vi "Charakterystyki.vi"() -> ()   [LabVIEW 2020]
uses:
  <vilib>/addons/Digital Filter Design/Analysis.llb/DFD Plot Freq Response (Linear-Spaced).vi
  <vilib>/addons/Digital Filter Design/NI_DigFilterLicensed.lvlib
panel:
  in  "stop":bool
  out "Charakterystyka fazowa":cluster{"f0":dbl, "df":dbl, "values":dbl[]}[](graph)
  out "Charakterystyka amplitudowa":cluster{"f0":dbl, "df":dbl, "values":dbl[]}[](graph)
  out "Charakterystyka fazowa":cluster{"f0":dbl, "df":dbl, "values":dbl[]}[](graph)
  out "Charakterystyka amplitudowa":cluster{"f0":dbl, "df":dbl, "values":dbl[]}[](graph)
  out "Charakterystyka fazowa":cluster{"f0":dbl, "df":dbl, "values":dbl[]}[](graph)
  out "Charakterystyka amplitudowa":cluster{"f0":dbl, "df":dbl, "values":dbl[]}[](graph)
  # "Filtr Butterwortha"
  # "Filtr Czebyszewa"
  # "Filtr Bessela"
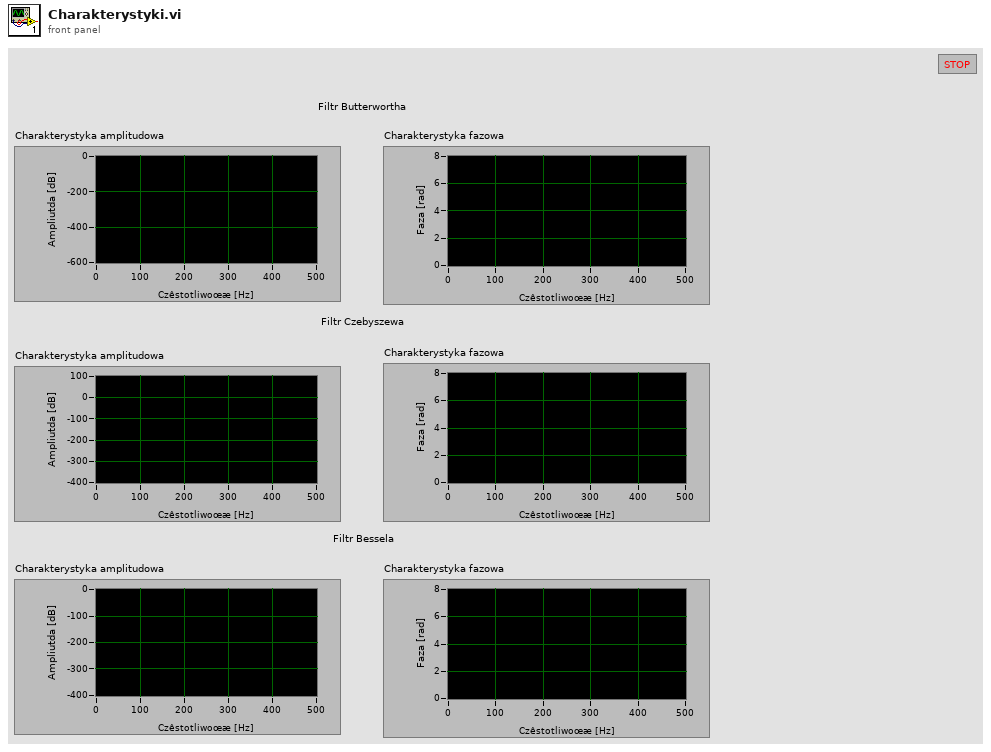
[diagram p1: front panel]
types:
  T1 = enum16{"Lowpass", "Highpass", "Bandpass", "Bandstop"}
  T2 = typedef "NI_DigFilterLicensed.lvlib/DFD Filter Obj.ctl" = cluster{"mSRate_Fs":dbl, "mSRate_Version":string, "mSRate_Comments":string, "mSRate_OrgCoef":T3, "mSRate_CurCoef":T3, "mSRate_Quantized?":bool, "mSRate_QCoef":T3, "mSRate_QSettings":T5[], "mSRate_Order":i32, "mSRate_Scaling":cluster{"mSRate_ScaleByPowerOf2?":bool, "mSRate_ScaleType":T7}}
  T3 = typedef "NI_DigFilterLicensed.lvlib/DFD Filter Coef.ctl" = cluster{"type":T4, "gain":dbl, "coef a (k)":dbl[], "coef b (v)":dbl[]}
  T4 = typedef "NI_DigFilterLicensed.lvlib/DFD Filter Structure Type Selector.ctl" = enum16{"Undefined", "FIR Direct Form", "FIR Direct Form Transposed", "FIR Symmetric", "FIR Antisymmetric", "IIR Direct Form I", "IIR Direct Form I Transposed", "IIR Direct Form II", "IIR Direct Form II Transposed", "IIR Cascaded Second Order Sections Form I", "IIR Cascaded Second Order Sections Form I Transposed", "IIR Cascaded Second Order Sections Form II", "IIR Cascaded Second Order Sections Form II Transposed", "Lattice Allpass (basic sections)", "Lattice Allpass (one multiplier sections)", "Lattice Allpass (normalized sections)", "Lattice AR (basic sections)", "Lattice AR (one multiplier sections)", "Lattice AR (normalized sections)", "Lattice MA (minimum phase)", "Lattice MA (maximum phase)", "Lattice ARMA (basic sections)", "Lattice ARMA (one multiplier sections)", "Lattice ARMA (normalized sections)"}
  T5 = typedef "NI_DigFilterLicensed.lvlib/dfd_Internal Quantization Settings.ctl" = cluster{"source":T6, "wl":i16, "iwl":i16, "overflow mode":enum16{"Saturation", "Wrap"}, "rounding mode":enum16{"Nearest", "Truncation"}, "signed?":bool}
  T6 = typedef "NI_DigFilterLicensed.lvlib/dfd_Internal Quantization Srcs.ctl" = u16
  T7 = typedef "NI_DigFilterLicensed.lvlib/DFD Coef Norm Type.ctl" = enum16{"No Norm", "Time Domain 1-Norm", "Time Domain 2-Norm", "Time Domain Inf-Norm"}
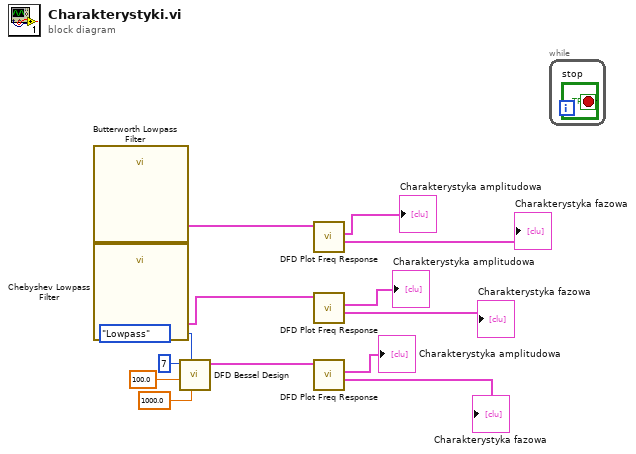
[diagram p0: block diagram]
diagram:
  n1 = call "Butterworth Lowpass Filter"() -> ("filter out"=w6:T2)  [unwired: 10 in, 1 out]
  n2 = call "Chebyshev Lowpass Filter"() -> ("filter out"=w5:T2)  [unwired: 10 in, 1 out]
  n3 = call <vilib>:"DFD Bessel Design.vi"("fs [Hz]"=1000.0, "filter type"=T1."Lowpass", "low cutoff freq [Hz]"=100.0, "order"=7) -> ("filter out"=w13:T2)  [unwired: 6 in, 1 out]
  n4 = call-poly <vilib>:"DFD Plot Freq Response.vi"("filter in"=w6) -> ("phase response"=→"Charakterystyka fazowa":cluster{"f0":dbl, "df":dbl, "values":dbl[]}[], "magnitude response"=→"Charakterystyka amplitudowa":cluster{"f0":dbl, "df":dbl, "values":dbl[]}[])  [unwired: 7 in, 2 out]
  n5 = call-poly <vilib>:"DFD Plot Freq Response.vi"("filter in"=w5) -> ("phase response"=→"Charakterystyka fazowa":cluster{"f0":dbl, "df":dbl, "values":dbl[]}[], "magnitude response"=→"Charakterystyka amplitudowa":cluster{"f0":dbl, "df":dbl, "values":dbl[]}[])  [unwired: 7 in, 2 out]
  n6 = call-poly <vilib>:"DFD Plot Freq Response.vi"("filter in"=w13) -> ("phase response"=→"Charakterystyka fazowa":cluster{"f0":dbl, "df":dbl, "values":dbl[]}[], "magnitude response"=→"Charakterystyka amplitudowa":cluster{"f0":dbl, "df":dbl, "values":dbl[]}[])  [unwired: 7 in, 2 out]
  n7 = while {
    stop <- "stop" stop-if-true
  }
